vi "errorInfo.vi"(5 "error in (no error)":errorcluster) -> (14 "HGF_Error":T2, 16 "HGF_Severity":T1=enum."Error", 19 "error out":errorcluster)   [LabVIEW 2012, in "HGF_Auxiliary.lvlib"]
doc: "This VI extracts from an HGF error cluster the error code and severity."
uses:
  HGF_Auxiliary.lvlib
  ErrorCode.ctl
  Severity.ctl
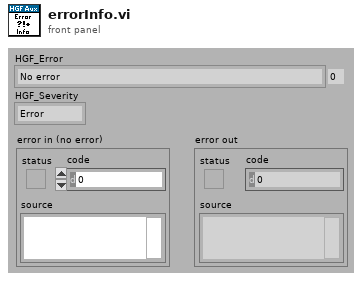
[diagram p1: front panel]
types:
  T1 = typedef "HGF_Auxiliary.lvlib/Severity.ctl" = enum16{"Info", "Warning", "Fault", "Error", "Fatal"}
  T2 = typedef "HGF_Auxiliary.lvlib/ErrorCode.ctl" = enum32{"No error", "Function not supported.", "This VI is for friends only.", "Reference object aready exisits.", "Parameter out of range.", "Not a rendezvous.", "Invalid notifier reference.", "Invalid queue reference.", "Self-Test not supported.", "Reset not supported.", "IDN query not supported.", "Error query not supported.", "Incorrect addressee.", "Object already exists.", "No class name specified", "Driver not supported", "Attribute is not writable"}
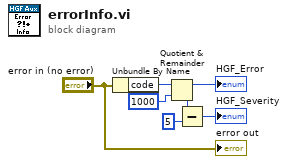
[diagram p0: block diagram]
diagram:
  n1 = Unbundle By Name("error in (no error)") -> ("code"=w4:i32)
  n2 = Quotient & Remainder(x=w4, y=1000) -> (x-y*floor(x/y)=→"HGF_Error":i32, floor(x/y)=w6:i32)
  n3 = Subtract(x=w6, y=5) -> (x-y=→"HGF_Severity":i32)
  "error out" <- "error in (no error)"
